vi "Oscilloscopee.vi"() -> ()   [LabVIEW 2020]
uses:
  <vilib>/Utility/miscctls.llb/LVRangeTypeDef.ctl
panel:
  in  "DC":dbl(knob) scale=0.0..10.0
  in  "V/div":dbl(knob) scale=0.0..10.0
  in  "stop":bool
  in  "Time / div":dbl(knob) scale=0.0..10.0
  out "Waveform Graph":waveform(dbl)(graph)
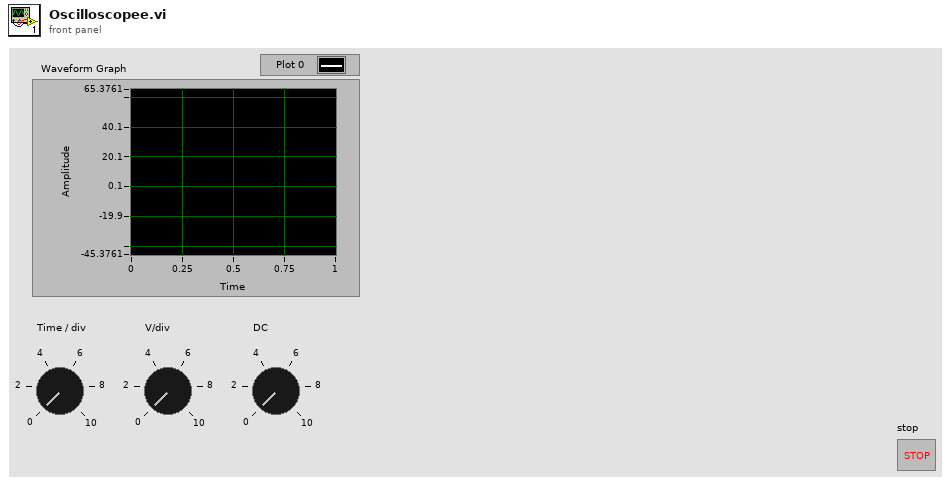
[diagram p1: front panel]
types:
  T1 = typedef "LVRangeTypeDef.ctl" = cluster{"Minimum":dbl, "Maximum":dbl, "Increment":dbl, "Minor Increment":dbl, "Start":dbl}
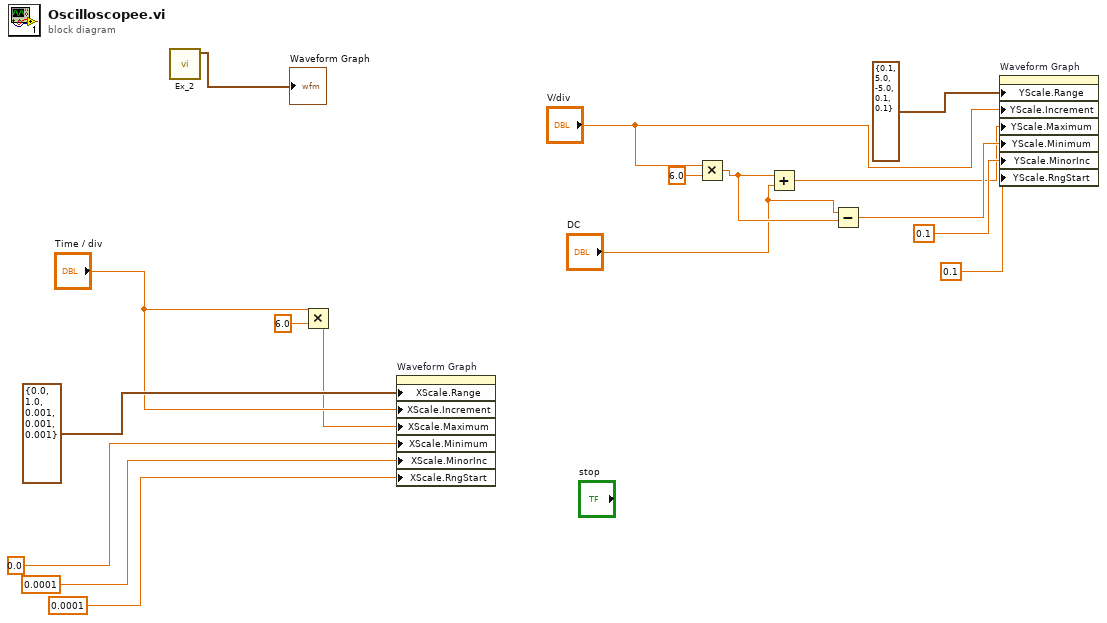
[diagram p0: block diagram]
diagram:
  n1 = call "Ex_2.vi"() -> ("Waveform Graph 2"=→"Waveform Graph":waveform(dbl))  [unwired: 11 in]
  n2 = Multiply(x="Time / div", y=6.0) -> (x*y=w3:dbl)
  n3 = property on="Waveform Graph" class="WFGraph (strict)"("XScale.Range"=T1 {"Minimum"=0.0, "Maximum"=1.0, "Increment"=0.001, "Minor Increment"=0.001, "Start"=0.001} ("X Scale.Range"), "XScale.Increment"="Time / div", "XScale.Maximum"=w3, "XScale.Minimum"=0.0 ("X Scale.Range:Minimum"), "XScale.MinorInc"=0.0001 ("X Scale.Range:Minor Increment"), "XScale.RngStart"=0.0001 ("X Scale.Range:Start")) -> ()  [unwired: 2 in, 2 out]
  n4 = Multiply(x="V/div", y=6.0) -> (x*y=w8:dbl)
  n5 = Add(x=w8, y="DC") -> (x+y=w1:dbl)
  n6 = Subtract(x="DC", y=w8) -> (x-y=w6:dbl)
  n7 = property on="Waveform Graph" class="WFGraph (strict)"("YScale.Range"=T1 {"Minimum"=0.1, "Maximum"=5.0, "Increment"=-5.0, "Minor Increment"=0.1, "Start"=0.1} ("Y Scale.Range"), "YScale.Increment"="V/div", "YScale.Maximum"=w1, "YScale.Minimum"=w6, "YScale.MinorInc"=0.1 ("Y Scale.Range:Minor Increment"), "YScale.RngStart"=0.1 ("Y Scale.Range:Start")) -> ()  [unwired: 2 in, 2 out]
